vi "_readUntilWhitespaceOrSeparator.vi"(8 "error in (no error)":errorcluster, 11 "tJSONParser in":refnum<class "tJSONParser.lvclass">) -> (0 "error out":errorcluster, 2 "String Out":string, 3 "tJSONParser out":refnum<class "tJSONParser.lvclass">)   [LabVIEW 2013, in "JSON.lvlib" / "tJSONParser.lvclass"]
doc: "Reads and returns all tokens up to, but not including, whitespace, '}', ']', or ','. This also validates that the string being returned is a valid number, boolean, or null value."
uses:
  tJSONParser.lvclass
  tJSONParser.lvclass/tJSONParser.ctl
  _tokenType.ctl
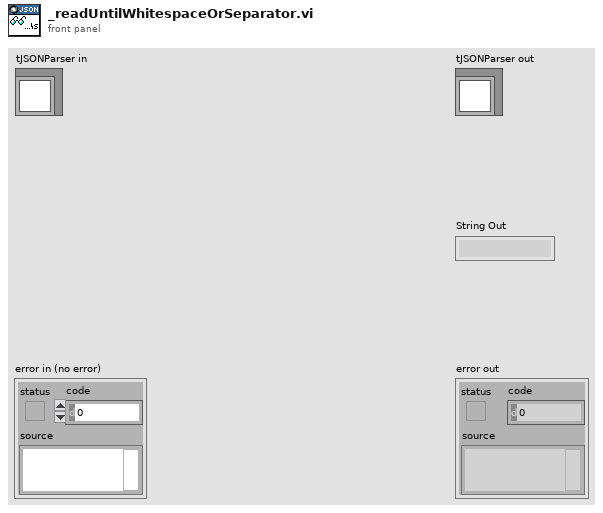
[diagram p1: front panel]
types:
  T1 = typedef "JSON.lvlib/tJSONParser.lvclass/_tokenType.ctl" = enum16{"Object Begin", "Object End", "Array Begin", "Array End", "String Delimeter", "Forward Slash", "Number", "Boolean", "Null", "Object Or Array Separator", "Pair Separator", "End Of File", "Asterisk", "Backward Slash", "Other"}
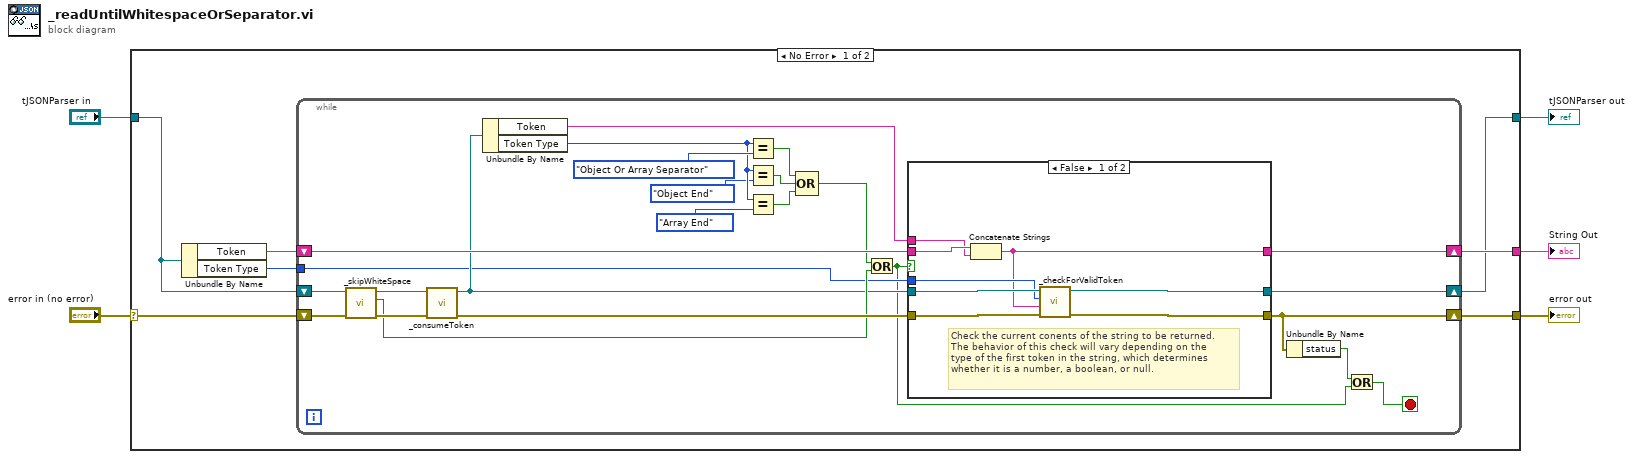
[diagram p0: block diagram]
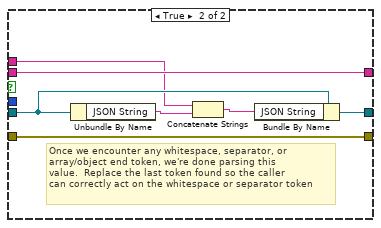
[diagram p2: hidden frame]
diagram:
  n1 = case shown="No Error" "error in (no error)" {
    selector: "error in (no error)" -> [w12 w53]
    tunnel: [w11 w53] -> w4
    tunnel: [w7 w52] -> w2
    tunnel: "tJSONParser in" -> [w10 w52]
    tunnel: [w8 _] -> w1
    frame No Error {
      n2 = Unbundle By Name(w10) -> ("Token"=w9:string, "Token Type"=w6:T1)
      n3 = while {
        shift-right: [w16] -> w11
        shift-left: w12 -> [w31]
        shift-right: [w36] -> w7
        shift-left: w10 -> [w32]
        shift-right: [w34] -> w8
        shift-left: w9 -> [w35]
        tunnel: w6 -> [w17]
        stop <- w13 stop-if-true
        n4 = call "_skipWhiteSpace.vi"("error in (no error)"=w31, "JSON Parser In"=w32) -> ("error out"=w29:errorcluster, "White Space Found?"=w21:bool, "JSON Parser Out"=w30:refnum<class "tJSONParser.lvclass">)  [unwired: 5 in, 2 out]
        n5 = call "_consumeToken.vi"("error in (no error)"=w29, "JSON Parser In"=w30) -> ("error out"=w28:errorcluster, "JSON Parser Out"=w18:refnum<class "tJSONParser.lvclass">)  [unwired: 8 in]
        n6 = Unbundle By Name(w18) -> ("Token"=w19:string, "Token Type"=w27:T1)
        n7 = Equal?(x=w27, y=_tokenType."Object Or Array Separator") -> (x = y?=w22:bool)
        n8 = Equal?(x=w27, y=_tokenType."Object End") -> (x = y?=w24:bool)
        n9 = Equal?(x=w27, y=_tokenType."Array End") -> (x = y?=w23:bool)
        n10 = Compound Arithmetic op=OR(w22, w24, w23) -> (w20:bool)
        n11 = Or(x=w20, y=w21) -> (x .or. y?=w14:bool)
        n12 = case shown="False" w14 {
          tunnel: [w42 w51] -> w16
          tunnel: w28 -> [w43 w51]
          tunnel: w18 -> [w41 w48]
          tunnel: [w40 w46] -> w36
          tunnel: w35 -> [w44 w47]
          tunnel: [w37 w47] -> w34
          tunnel: w19 -> [w39 w45]
          tunnel: w17 -> [w38 _]
          frame False {
            # "Check the current conents of the string to be returned.\nThe behavior of this check will vary depending on the \ntype of the first token in the string, which determines\nwhether it is a number, a boolean, or null."
            n13 = Concatenate Strings(w44, w39) -> (w37:string)
            n14 = call "_checkForValidToken.vi"("error in (no error)"=w43, "String"=w37, "Token Type"=w38, "tJSONParser in"=w41) -> ("error out"=w42:errorcluster, "tJSONParser out"=w40:refnum<class "tJSONParser.lvclass">)  [unwired: 6 in]
          }
          frame True {
            # "Once we encounter any whitespace, separator, or \narray/object end token, we're done parsing this \nvalue.  Replace the last token found so the caller\ncan correctly act on the whitespace or separator token"
            n15 = Unbundle By Name(w48) -> ("JSON String"=w50:string)
            n16 = Concatenate Strings(w45, w50) -> (w49:string)
            n17 = Bundle By Name(cluster=w48, "JSON String"=w49) -> (w46:refnum<class "tJSONParser.lvclass">)
          }
        }
        n18 = Unbundle By Name(w16) -> ("status"=w15:bool)
        n19 = Or(x=w15, y=w14) -> (x .or. y?=w13:bool)
      }
    }
    frame Error {
    }
  }
  "error out" <- w4
  "tJSONParser out" <- w2
  "String Out" <- w1
